vi "Destroy.vi"(0 "reference in":refnum<class "Notification Controller.lvclass">, 5 "error in (no error)":errorcluster) -> (14 "reference out":refnum<class "Notification Controller.lvclass">, 19 "error out":errorcluster)   [LabVIEW 2015, in "Notification Controller.lvclass"]
doc: "Destructor."
uses:
  Notification Controller.lvclass
  APP/trackingNotification_class/trackingNotification.lvclass
  APP/itemsNotification_class/itemsNotification.lvclass
  <vilib>/addons/_AddQ/G#Object/G#Object.lvclass
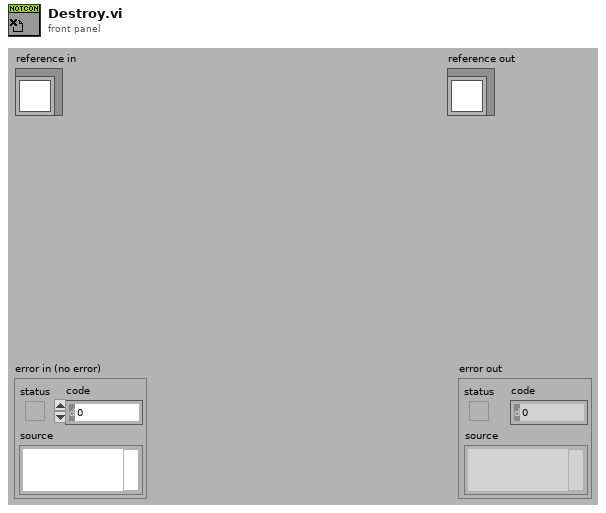
[diagram p1: front panel]
types:
  T1 = typedef "Notification Controller.lvclass/ObjectAttributes.ctl" = cluster{"MyAttribute":dbl, "items_data":string[][][], "items_notification_refs":refnum<class "itemsNotification.lvclass">[], "notifications_data_items":string[][], "items_nots?":bool, "devices_controller_ref":refnum<class "Devices Controller.lvclass">, "onlineUpdate":timestamp, "notController?":bool, "tracking_notification_ref":refnum<class "trackingNotification.lvclass">, "notifications_data_tracking":string[][], "tracking_parts_data":string[][], "tracking_nots?":bool, "index_tracking_not":i32[], "file_controller_ref":refnum<class "File Controller.lvclass">}
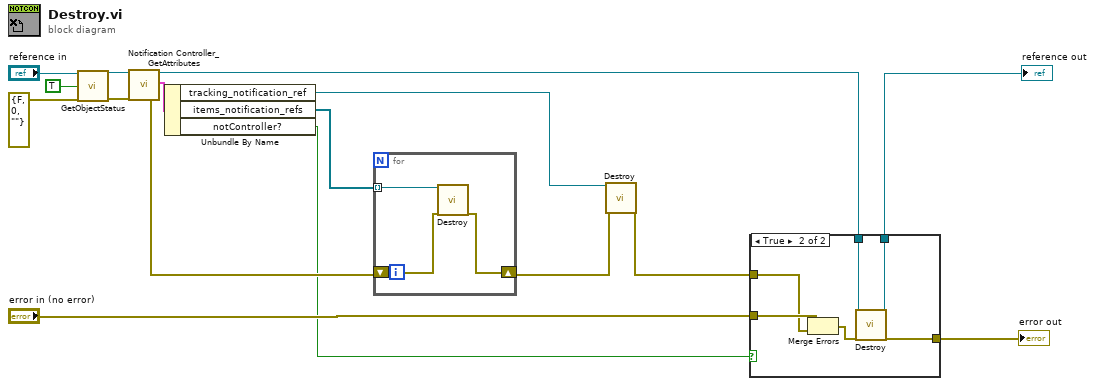
[diagram p0: block diagram]
diagram:
  n1 = call-dynamic "GetObjectStatus.vi"("reference in"="reference in", "simple info (F)"=TRUE ("simple info"), "error in (no error)"=errorcluster {"status"=FALSE, "code"=0, "source"=""}) -> ("reference out"=w11:refnum<class "Notification Controller.lvclass">, "error out"=w12:errorcluster)  [unwired: 5 in, 10 out]
  n2 = call "Notification Controller_GetAttributes.vi"("reference in"=w11, "error in (no error)"=w12) -> ("reference out"=w10:refnum<class "Notification Controller.lvclass">, "attributes"=w4:T1, "error out"=w6:errorcluster)  [unwired: 14 in, 1 out]
  n3 = Unbundle By Name(w4) -> ("tracking_notification_ref"=w3:refnum<class "trackingNotification.lvclass">, "items_notification_refs"=w7:refnum<class "itemsNotification.lvclass">[], "notController?"=w5:bool)
  n4 = for {
    tunnel: w7 -> [w19] mode=indexing
    shift-right: [w17] -> w2
    shift-left: w6 -> [w18]
    n5 = call-dynamic "Destroy.vi"("reference in"=w19, "error in (no error)"=w18) -> ("error out"=w17:errorcluster)  [unwired: 16 in, 1 out]
  }
  n6 = call-dynamic "Destroy.vi"("reference in"=w3, "error in (no error)"=w2) -> ("error out"=w1:errorcluster)  [unwired: 16 in, 1 out]
  n7 = case shown="True" w5 {
    tunnel: "error in (no error)" -> [_ w27]
    tunnel: w10 -> [w20 w25]
    tunnel: [w21 w24] -> w9
    tunnel: [w20 w23] -> w8
    tunnel: w1 -> [w21 w22]
    frame False {
    }
    frame True {
      n8 = Merge Errors(w27, w22) -> (w26:errorcluster)
      n9 = call-parent "Destroy.vi"("reference in"=w25, "error in (no error)"=w26) -> ("reference out"=w23:refnum<class "Notification Controller.lvclass">, "error out"=w24:errorcluster)  [unwired: 16 in]
    }
  }
  "error out" <- w9
  "reference out" <- w8
